vi "Z900_navX_SERIAL_CapturePacket.vi"(11 "Buffer":string) -> (0 "Packet Size":i32, 1 "Packet Located":bool, 2 "Packet":string, 3 "Buffer":string)   [LabVIEW 2025]
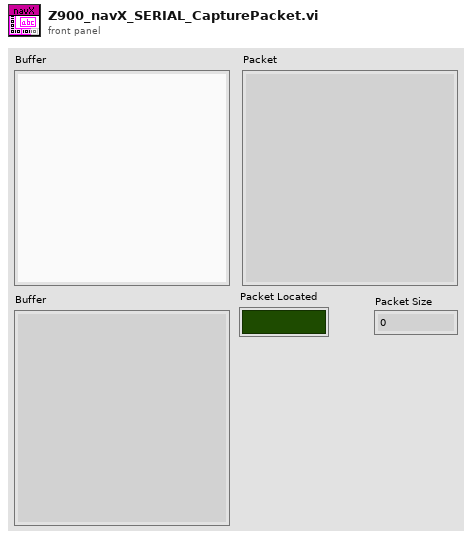
[diagram p1: front panel]
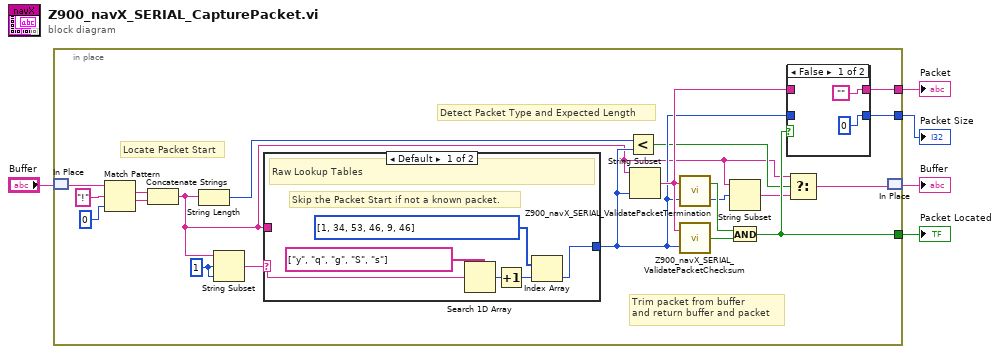
[diagram p0: block diagram]
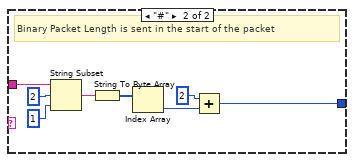
[diagram p2: hidden frame]
diagram:
  n1 = in-place {
    in-place-border: [w25] -> w5
    in-place-border: [w24] -> w4
    in-place-border: [w22] -> w3
    w21 = 1 ("length (rest)")
    # "Locate Packet Start"
    # "Trim packet from buffer\nand return buffer and packet"
    # "Detect Packet Type and Expected Length"
    n2 = in-place-match #1("Buffer") -> (w12:string)
    n3 = Match Pattern(string=w12, regular expression="!" ("Packet Start Char"), offset (0)=0 ("offset past match")) -> (match substring=w16:string, after substring=w15:string)  [unwired: 2 out]
    n4 = Concatenate Strings(w16, w15) -> (w8:string)
    n5 = String Length(string=w8) -> (length=w11:i32)
    n6 = String Subset(string=w8, offset (0)=w21, length (rest)=w21) -> (substring=w20:string)
    n7 = case shown="Default" w20 {
      selector: w20 -> [w27 _]
      tunnel: [w28 w35] -> w10
      tunnel: w8 -> [_ w33]
      frame Default {
        # "Skip the Packet Start if not a known packet."
        # "Raw Lookup Tables"
        n8 = Search 1D Array(1D array=string[] ["y", "q", "g", "S", "s"], element=w27) -> (index of element=w29:i32)  [unwired: 1 in]
        n9 = Increment(x=w29) -> (x+1=w26:i32)
        n10 = Index Array(array=i32[] [1, 34, 53, 46, 9, 46], index=w26) -> (element=w28:i32)
      }
      frame "#" {
        # "Binary Packet Length is sent in the start of the packet"
        n11 = String Subset(string=w33, offset (0)=2, length (rest)=1 ("length (rest)")) -> (substring=w34:string)
        n12 = String To Byte Array(string=w34) -> (unsigned byte array=w37:u8[])
        n13 = Index Array(array=w37) -> (element=w38:u8)  [unwired: 1 in]
        n14 = Add(x=u8 2 ("y"), y=w38) -> (x+y=w35:u8)
      }
    }
    n15 = Less?(x=w11, y=w10) -> (x < y?=w9:bool)
    n16 = String Subset(string=w8, length (rest)=w10) -> (substring=w23:string)  [unwired: 1 in]
    n17 = call "Z900_navX_SERIAL_ValidatePacketTermination.vi"("Expected Packet Length"=w10, "Buffer"=w23) -> ("Packet Termination Offset"=w17:i32, "Packet Valid"=w18:bool)
    n18 = call "Z900_navX_SERIAL_ValidatePacketChecksum.vi"("Expected Packet Length"=w10, "Buffer"=w23) -> ("Packet Valid"=w19:bool)
    n19 = String Subset(string=w8, offset (0)=w17) -> (substring=w7:string)  [unwired: 1 in]
    n20 = And(x=w18, y=w19) -> (x .and. y?=w25:bool)
    n21 = case shown="False" w25 {
      tunnel: ["" w43] -> w24
      tunnel: w23 -> [_ w43]
      tunnel: [0 w42] -> w22
      tunnel: w10 -> [_ w42]
      frame False {
      }
      frame True {
      }
    }
    n22 = Select(t=w8, s=w9, f=w7) -> (s? t:f=w6:string)
    n23 = in-place-match #1(w6) -> (→"Buffer":string)
  }
  "Packet" <- w4
  "Packet Located" <- w5
  "Packet Size" <- w3
